vi "Delete.vi"(10 "Key":string, 11 "Dictionary in":variant) -> (2 "found":bool, 3 "Dictionary out":variant)   [LabVIEW 2013, in "Dictionary.lvlib"]
doc: "Delete value from dictionary with the passed in key."
uses:
  Dictionary.lvlib
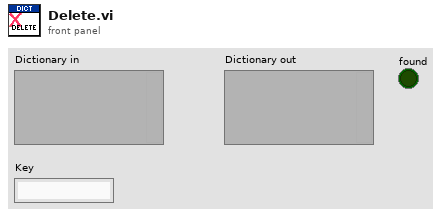
[diagram p1: front panel]
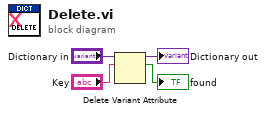
[diagram p0: block diagram]
diagram:
  n1 = Delete Variant Attribute(6:"Key", 7:"Dictionary in") -> (2:→"found":bool, 3:→"Dictionary out":variant)  [unwired: 1 in, 1 out]
